vi "Fct_Write_On_File.vi"(11 "Chaîne":string) -> (0 "sortie d'erreur":errorcluster)   [LabVIEW 2017]
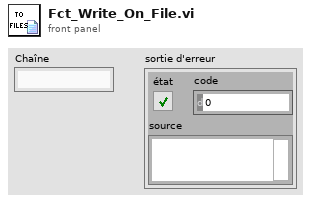
[diagram p1: front panel]
types:
  T1 = enum16{"open", "replace", "create", "open or create", "replace or create", "replace or create with confirmation"}
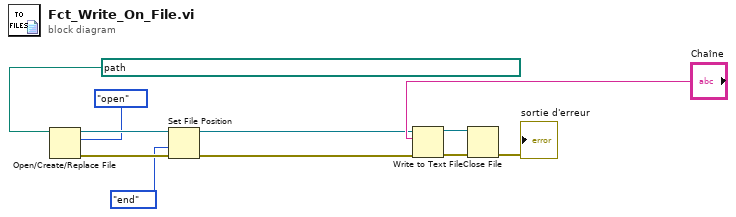
[diagram p0: block diagram]
diagram:
  n1 = Open/Create/Replace File(file path (use dialog)=path "E:/ESIGELEC/Phase 2/Instrumentation et systèmes/Station météo/Alarmes.txt" ("chemin du fichier (utiliser une boîte de dialogue)"), operation (0:open)=T1."open" ("opération (0 : open)")) -> (refnum out=w3:refnum<file>, error out=w5:errorcluster)  [unwired: 4 in, 1 out]
  n2 = Set File Position(refnum=w3, from (0:start)=enum16{"start", "end", "current"}."end" ("à partir de (0 : start)"), error in=w5) -> (refnum out=w7:refnum<file>, error out=w9:errorcluster)  [unwired: 1 in]
  n3 = Write to Text File(file (use dialog)=w7, text="Chaîne", error in=w9) -> (refnum out=w6:refnum<file>, error out=w10:errorcluster)  [unwired: 1 in, 1 out]
  n4 = Close File(refnum=w6, error in=w10) -> (error out=→"sortie d'erreur":errorcluster)  [unwired: 1 out]
